vi "串口配置.vi"() -> ()   [LabVIEW 2016, in "数据传输系统.lvlib"]
panel:
  in  "baud rate":u32=9600 caption="波特率"
  in  "VISA resource name":refnum<visa-resource-name> caption="VISA资源名称"
  # "串口配置"
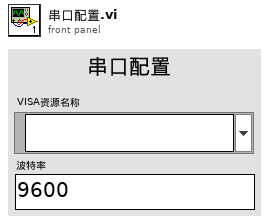
[diagram p1: front panel]
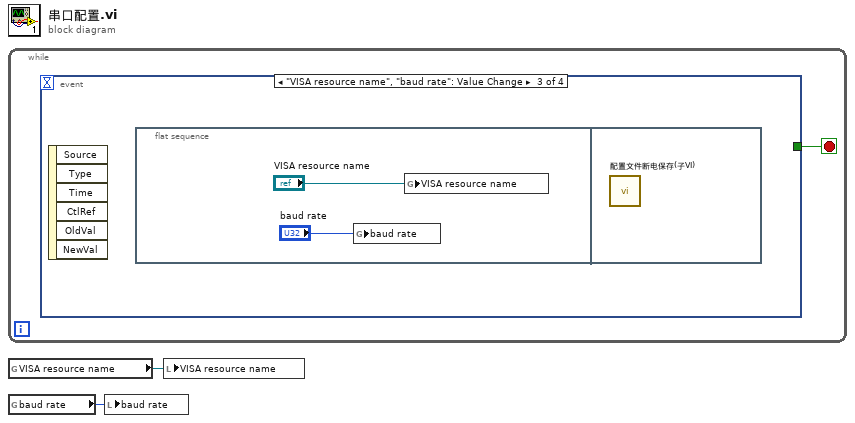
[diagram p0: block diagram]
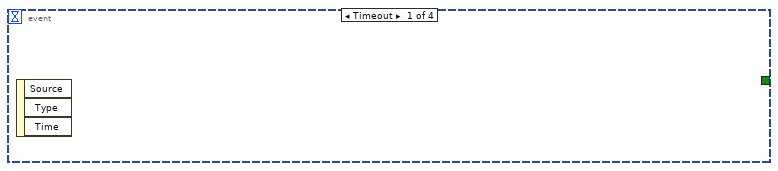
[diagram p2: hidden frame]
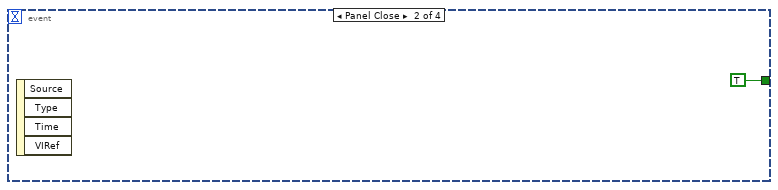
[diagram p3: hidden frame]
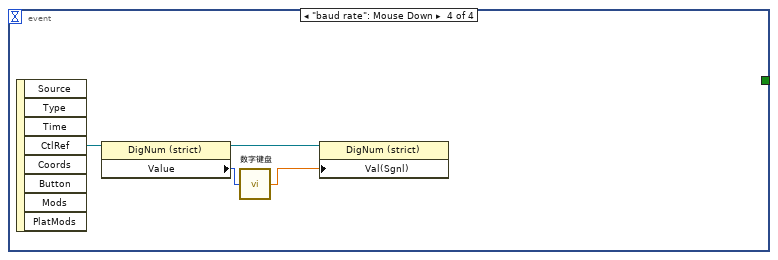
[diagram p4: hidden frame]
diagram:
  n1 = while {
    stop <- w3 stop-if-true
    n2 = event shown="[2] \"VISA resource name\", \"baud rate\": Value Change" {
      selector: _ -> [_ _ _ _]
      dyn-events: _ -> [_ _ _ _]
      timeout: _ -> [_ _ _ _]
      tunnel: [_ TRUE _ _] -> w3
      event Timeout {
        n3 = event-data() -> ()  [unwired: 1 in, 3 out]
      }
      event Panel Close {
        n4 = event-data() -> ()  [unwired: 1 in, 4 out]
      }
      event "VISA resource name", "baud rate": Value Change {
        n5 = event-data() -> ()  [unwired: 1 in, 6 out]
        n6 = flat-sequence {
          frame #0 {
            n7 = global write "断电保存全局.vi" "baud rate"("baud rate") -> ()
            n8 = global write "断电保存全局.vi" "VISA resource name"("VISA resource name") -> ()
          }
          frame #1 {
            n9 = call "配置文件断电保存(子VI).vi"() -> ()  [unwired: 12 in]
          }
        }
      }
      event "baud rate": Mouse Down {
        n10 = event-data() -> ("CtlRef"=w10:refnum<vi>)  [unwired: 1 in, 7 out]
        n11 = property class="DigNum (strict)"(reference=w10) -> (reference out=w9:refnum<vi>, "Value"=w8:u32)  [unwired: 1 in, 1 out]
        n12 = call "数字键盘.vi"("OldNumber"=w8) -> ("NewNumber"=w7:sgl)
        n13 = property class="DigNum (strict)"(reference=w9, "Val(Sgnl)"=w7) -> ()  [unwired: 1 in, 2 out]
      }
    }
  }
  n14 = global read "断电保存全局.vi" "VISA resource name"() -> (w2:refnum<visa-resource-name>)
  n15 = global read "断电保存全局.vi" "baud rate"() -> (w1:u32)
  n16 = local write "baud rate"(w1) -> ()
  n17 = local write "VISA resource name"(w2) -> ()
